vi "Integer.vi"(7 "data type of variable":i32, 8 "error in":errorcluster, 10 "variable name":string, 11 "pipe in":T1) -> (0 "error out":errorcluster, 2 "value":i32, 3 "pipe out":T1)   [LabVIEW 2013, in "GOLPI library.lvlib"]
uses:
  GOLPI library.lvlib
  LV Process.lvlibp/Pipe Handle.ctl
  Globals.vi
  <vilib>/Utility/error.llb/Error Cluster From Error Code.vi
  <vilib>/regexp/Match Regular Expression.xnode
  <vilib>/ErrorRing/Error Ring.xnode
  LV Process.lvlibp
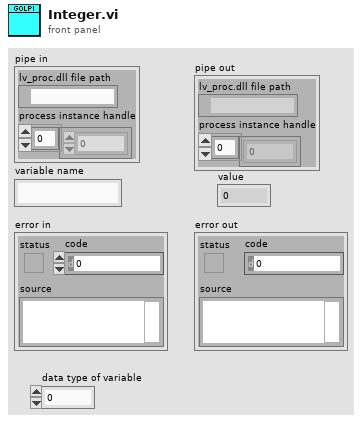
[diagram p1: front panel]
types:
  T1 = typedef "LV Process.lvlibp/Pipe Handle.ctl" = cluster{"lv_proc.dll file path":path, "process instance handle":u32[]}
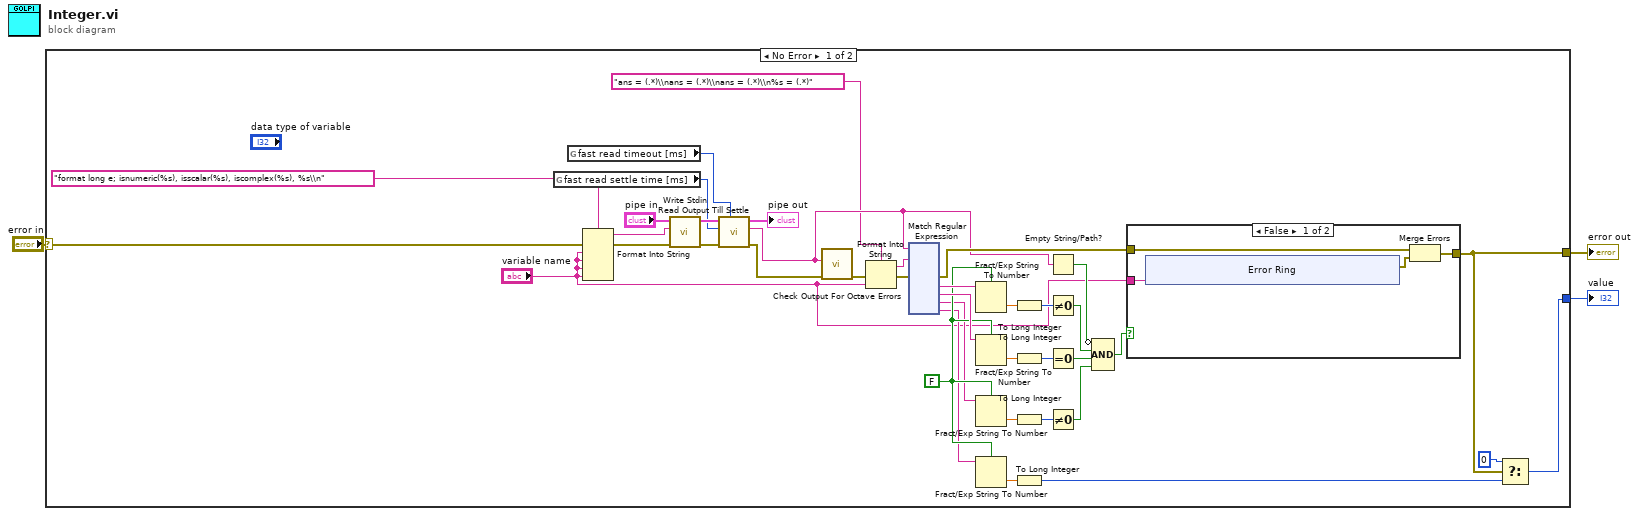
[diagram p0: block diagram]
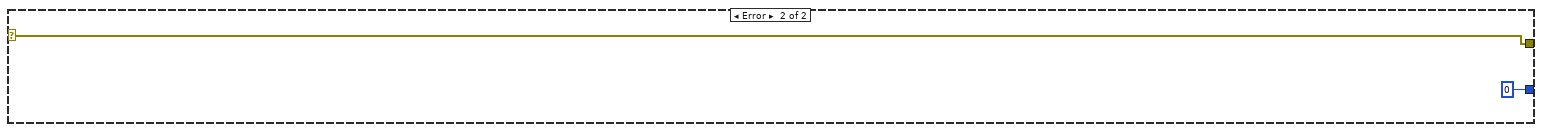
[diagram p3: hidden frame]
diagram:
  n1 = case shown="No Error" "error in" {
    selector: "error in" -> [w10 w174]
    tunnel: [w13 0 ("t")] -> w3
    tunnel: [w12 w174] -> w2
    frame No Error {
      w33 = FALSE ("use system decimal point (T)")
      n2 = global read "Globals.vi" "fast read settle time [ms]"() -> (w22:u32)
      n3 = global read "Globals.vi" "fast read timeout [ms]"() -> (w21:u32)
      n4 = Format Into String(format string="format long e; isnumeric(%s), isscalar(%s), iscomplex(%s), %s\\n", error in=w10, "variable name", "variable name", "variable name", "variable name") -> (resulting string=w35:string, error out=w9:errorcluster)  [unwired: 1 in]
      n5 = call "Write Stdin.vi"("error in"=w9, "write buffer"=w35, "pipe in"="pipe in") -> ("error out"=w23:errorcluster, "pipe out"=w41:T1)  [unwired: 6 in, 1 out]
      n6 = call "Read Output Till Settle.vi"("timeout [ms]"=w21, "error in"=w23, "settled for [ms]"=w22, "pipe in"=w41) -> ("error out"=w25:errorcluster, "read buffer"=w11:string, "pipe out"=→"pipe out":T1)  [unwired: 4 in, 1 out]
      n7 = call "Check Output For Octave Errors.vi"("error in"=w25, "read buffer"=w11) -> ("error out"=w6:errorcluster)  [unwired: 9 in]
      n8 = Format Into String(format string="ans = (.*)\\nans = (.*)\\nans = (.*)\\n%s = (.*)" ("regular expression"), error in=w6, "variable name") -> (resulting string=w7:string, error out=w5:errorcluster)  [unwired: 1 in]
      n9 = xnode "Match Regular Expression"("input string"=w11, "regular expression"=w7, "error in"=w5) -> ("error out"=w24:errorcluster, "submatch 1"=w39:string, "submatch 2"=w34:string, "submatch 3"=w32:string, "submatch 4"=w31:string)  [unwired: 3 in, 4 out]
      n10 = Fract/Exp String To Number(use system decimal point (T)=w33, string=w39) -> (number=w38:dbl)  [unwired: 2 in, 1 out]
      n11 = Fract/Exp String To Number(use system decimal point (T)=w33, string=w34) -> (number=w28:dbl)  [unwired: 2 in, 1 out]
      n12 = Fract/Exp String To Number(use system decimal point (T)=w33, string=w32) -> (number=w29:dbl)  [unwired: 2 in, 1 out]
      n13 = Fract/Exp String To Number(use system decimal point (T)=w33, string=w31) -> (number=w30:dbl)  [unwired: 2 in, 1 out]
      n14 = To Long Integer(number=w38) -> (32bit integer=w37:i32)
      n15 = To Long Integer(number=w28) -> (32bit integer=w27:i32)
      n16 = To Long Integer(number=w29) -> (32bit integer=w26:i32)
      n17 = To Long Integer(number=w30) -> (32bit integer=w15:i32)
      n18 = Empty String/Path?(string/path=w11) -> (empty?=w17:bool)
      n19 = Not Equal To 0?(x=w37) -> (x != 0?=w20:bool)
      n20 = Equal To 0?(x=w27) -> (x = 0?=w19:bool)
      n21 = Not Equal To 0?(x=w26) -> (x != 0?=w18:bool)
      n22 = Compound Arithmetic op=AND(invert w17, w20, w19, w18) -> (w16:bool)
      n23 = case shown="False" w16 {
        tunnel: [w44 w54] -> w12
        tunnel: w24 -> [w45 w54]
        tunnel: "variable name" -> [w43 _]
        frame False {
          n24 = xnode "Error Ring"("parameter 0"=w43) -> ("error out"=w46:errorcluster)
          n25 = Merge Errors(w45, w46) -> (w44:errorcluster)
        }
        frame True {
        }
      }
      n26 = Select(t=0, s=w12, f=w15) -> (s? t:f=w13:i32)
    }
    frame Error {
    }
  }
  "value" <- w3
  "error out" <- w2
